vi "Set Closed Loop Fréq.vi"(8 "error in (no error)":errorcluster caption="entrée d'erreur (pas d'erreur)", 10 "frequency":u32, 11 "UI SA en entrée":refnum<class "UI SmarAct.lvclass">) -> (0 "error out":errorcluster caption="sortie d'erreur", 3 "UI SA en sortie":refnum<class "UI SmarAct.lvclass">)   [LabVIEW 2024, in "UI SmarAct.lvclass"]
uses:
  UI SmarAct.lvclass
  UI SmarAct.lvclass/UI SmarAct.ctl
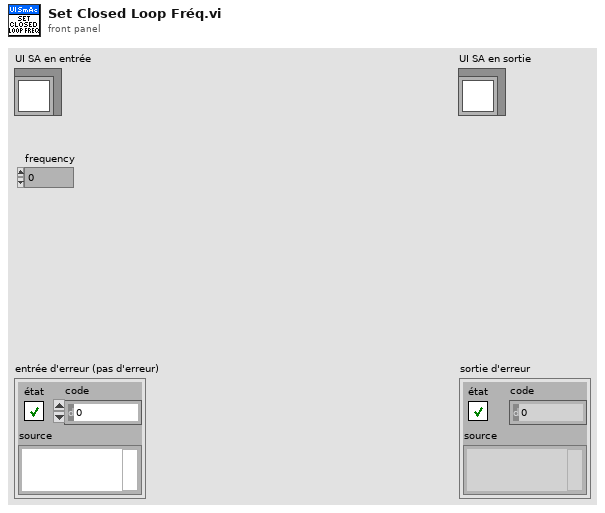
[diagram p1: front panel]
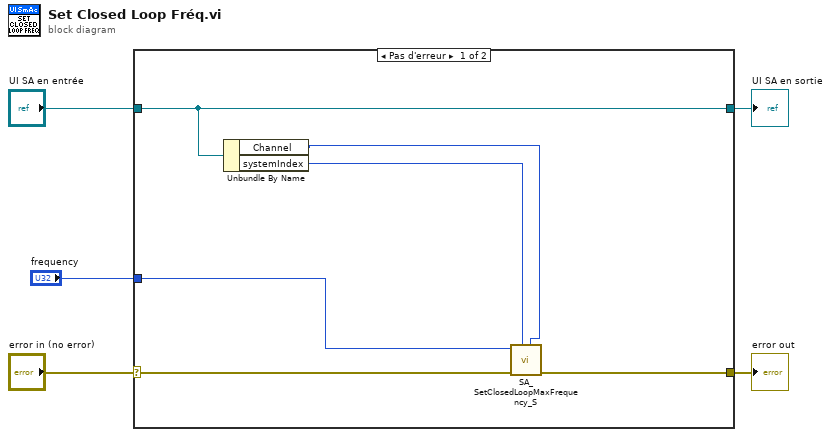
[diagram p0: block diagram]
diagram:
  n1 = case shown="Pas d'erreur" "error in (no error)" {
    selector: "error in (no error)" -> [w7 w13]
    tunnel: [w10 w13] -> w4
    tunnel: [w11 w12] -> w2
    tunnel: "UI SA en entrée" -> [w11 w12]
    tunnel: "frequency" -> [w6 _]
    frame No Error {
      n2 = Unbundle By Name(w11) -> ("Channel"=w8:u32, "systemIndex"=w9:u32)
      n3 = call <vilib>:"SA_SetClosedLoopMaxFrequency_S.vi"("channelIndex"=w8, "systemIndex"=w9, "error in (no error)"=w7, "frequency"=w6) -> ("error out"=w10:errorcluster)  [unwired: 7 in]
    }
    frame Error {
    }
  }
  "error out" <- w4
  "UI SA en sortie" <- w2
